vi "4155C SampleI Config SMUs.vi"(4 "error in (no error)":errorcluster, 7 "VISA resource name in":refnum<visa-resource-name>) -> (0 "error out":errorcluster, 3 "VISA Resource Name out":refnum<visa-resource-name>)   [LabVIEW 2016]
panel:
  in  "Gate Standby":bool
  in  "Drain Standby":bool
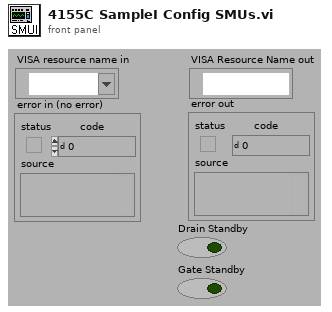
[diagram p1: front panel]
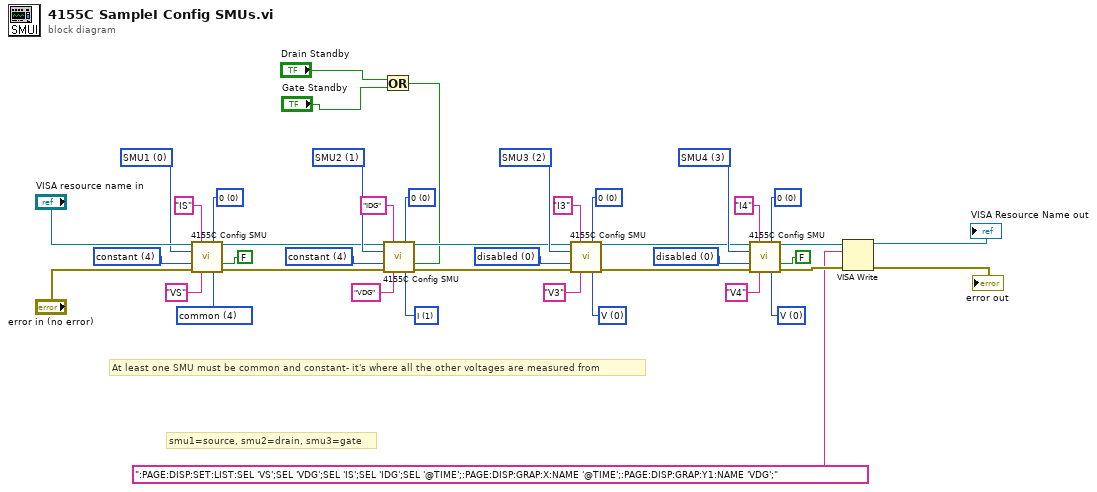
[diagram p0: block diagram]
diagram:
  w17 = u32 0 items=["V  ", "I  ", "V pulse  ", "I pulse  ", "  common  "] ("mode")
  w18 = u32 0 items=["0  ", "10K Ohms  ", "100K Ohms  ", "1M Ohms  "] ("series resistance *")
  w20 = u32 0 items=["disabled  ", "VAR1  ", "VAR2  ", "VAR1'  ", "constant  "] ("function")
  w21 = u32 3 items=["SMU1  ", "SMU2  ", "SMU3  ", "SMU4  ", "SMU5  ", "SMU6  "] ("unit to configure")
  w23 = u32 0 items=["V  ", "I  ", "V pulse  ", "I pulse  ", "  common  "] ("mode")
  w24 = u32 0 items=["0  ", "10K Ohms  ", "100K Ohms  ", "1M Ohms  "] ("series resistance *")
  w26 = u32 0 items=["disabled  ", "VAR1  ", "VAR2  ", "VAR1'  ", "constant  "] ("function")
  w27 = u32 2 items=["SMU1  ", "SMU2  ", "SMU3  ", "SMU4  ", "SMU5  ", "SMU6  "] ("unit to configure")
  w29 = u32 1 items=["V  ", "I  ", "V pulse  ", "I pulse  ", "  common  "] ("mode")
  w30 = u32 0 items=["0  ", "10K Ohms  ", "100K Ohms  ", "1M Ohms  "] ("series resistance *")
  w32 = u32 4 items=["disabled  ", "VAR1  ", "VAR2  ", "VAR1'  ", "constant  "] ("function")
  w33 = u32 1 items=["SMU1  ", "SMU2  ", "SMU3  ", "SMU4  ", "SMU5  ", "SMU6  "] ("unit to configure")
  w36 = u32 4 items=["V  ", "I  ", "V pulse  ", "I pulse  ", "  common  "] ("mode")
  w37 = u32 0 items=["0  ", "10K Ohms  ", "100K Ohms  ", "1M Ohms  "] ("series resistance *")
  w39 = u32 4 items=["disabled  ", "VAR1  ", "VAR2  ", "VAR1'  ", "constant  "] ("function")
  w40 = u32 0 items=["SMU1  ", "SMU2  ", "SMU3  ", "SMU4  ", "SMU5  ", "SMU6  "] ("unit to configure")
  # "smu1=source, smu2=drain, smu3=gate"
  # "At least one SMU must be common and constant- it's where all the other voltages are measured from"
  n1 = call "4155C Config SMU.vi"("VISA session"="VISA resource name in", "I name (max 6 chars)"="IS", "series resistance *"=w37, "unit to configure"=w40, "function"=w39, "standby"=FALSE, "error in (no error)"="error in (no error)", "V name (max 6 chars)"="VS", "mode"=w36) -> ("dup VISA resource name"=w14:refnum<visa-resource-name>, "error out"=w13:errorcluster)  [unwired: 5 in]
  n2 = Or(x="Drain Standby", y="Gate Standby") -> (x .or. y?=w1:bool)
  n3 = call "4155C Config SMU.vi"("VISA session"=w14, "I name (max 6 chars)"="IDG", "series resistance *"=w30, "unit to configure"=w33, "function"=w32, "standby"=w1, "error in (no error)"=w13, "V name (max 6 chars)"="VDG", "mode"=w29) -> ("dup VISA resource name"=w11:refnum<visa-resource-name>, "error out"=w12:errorcluster)  [unwired: 5 in]
  n4 = call "4155C Config SMU.vi"("VISA session"=w11, "I name (max 6 chars)"="I3", "series resistance *"=w24, "unit to configure"=w27, "function"=w26, "error in (no error)"=w12, "V name (max 6 chars)"="V3", "mode"=w23) -> ("dup VISA resource name"=w10:refnum<visa-resource-name>, "error out"=w9:errorcluster)  [unwired: 6 in]
  n5 = call "4155C Config SMU.vi"("VISA session"=w10, "I name (max 6 chars)"="I4", "series resistance *"=w18, "unit to configure"=w21, "function"=w20, "standby"=FALSE, "error in (no error)"=w9, "V name (max 6 chars)"="V4", "mode"=w17) -> ("dup VISA resource name"=w8:refnum<visa-resource-name>, "error out"=w7:errorcluster)  [unwired: 5 in]
  n6 = VISA Write(VISA resource name=w8, write buffer=":PAGE:DISP:SET:LIST:SEL 'VS';SEL 'VDG';SEL 'IS';SEL 'IDG';SEL '@TIME';:PAGE:DISP:GRAP:X:NAME '@TIME';:PAGE:DISP:GRAP:Y1:NAME 'VDG';" ("write buffer (\"\")"), error in (no error)=w7) -> (VISA resource name out=→"VISA Resource Name out":refnum<visa-resource-name>, error out=→"error out":errorcluster)  [unwired: 1 out]
